vi "Disabled.vi"(7 "Robot Mode":T2, 10 "Match Info":T1={"Autonomous Elapsed Seconds"=0.0, "TeleOp Elapsed Seconds"=0.0, "Disabled Elapsed Seconds"=0.0, "Visited Autonomous"=FALSE, "Visited TeleOp"=FALSE, "Visited Disabled"=FALSE, "Autonomous Settings"={"Autonomous Style"=enum."Independent", "VI Refnum"=refnum}}, 11 "Call Context":T3) -> ()   [LabVIEW 2014]
doc: "This VI is called each time a disabled packet is received from the DS. It is often used to prepare for the next robot mode, to calibrate sensors, etc."
uses:
  <vilib>/Rock Robotics/WPI/DriverStation/WPI_DriverStationDerivedRobotMode.ctl
  <vilib>/Rock Robotics/WPI/DriverStation/WPI_DriverStationRobotMode2.ctl
  <vilib>/Rock Robotics/WPI/DriverStation/WPI_DriverStationMatch Info.ctl
  Elevator System/Elevator System.lvlib
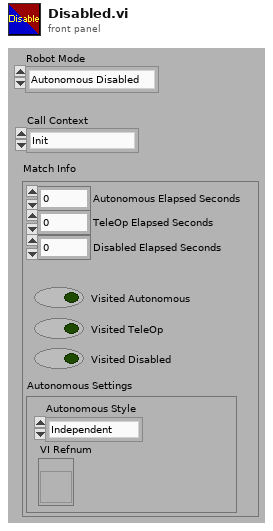
[diagram p1: front panel]
types:
  T1 = typedef "WPI_DriverStationMatch Info.ctl" = cluster{"Autonomous Elapsed Seconds":dbl, "TeleOp Elapsed Seconds":dbl, "Disabled Elapsed Seconds":dbl, "Visited Autonomous":bool, "Visited TeleOp":bool, "Visited Disabled":bool, "Autonomous Settings":cluster{"Autonomous Style":enum16{"Iterative", "Independent"}, "VI Refnum":refnum<vi>}}
  T2 = typedef "WPI_DriverStationRobotMode2.ctl" = enum16{"Autonomous Disabled", "Autonomous Enabled", "Teleop Disabled", "Teleop Enabled", "Disconnected", "Finish", "Test Disabled", "Test Enabled", "Emergency Stopped"}
  T3 = typedef "WPI_DriverStationDerivedRobotMode.ctl" = enum16{"Init", "Execute", "Stop"}
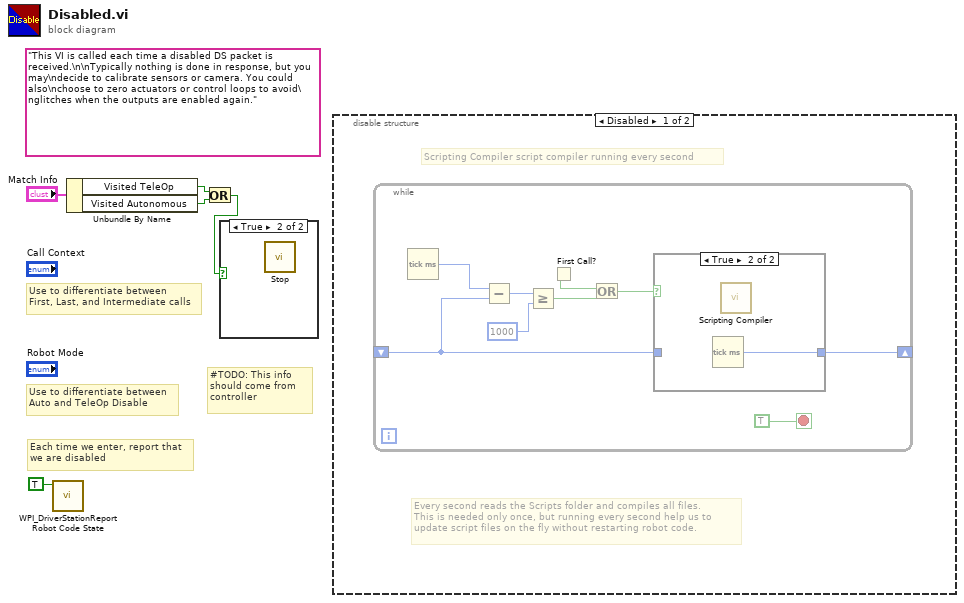
[diagram p0: block diagram]
diagram:
  (unwired) "This VI is called each time a disabled DS packet is received.\n\nTypically nothing is done in response, but you may\ndecide to calibrate sensors or camera. You could also\nchoose to zero actuators or control loops to avoid\nglitches when the outputs are enabled again."
  # "#TODO: This info\nshould come from \ncontroller"
  # "Each time we enter, report that\nwe are disabled"
  # "Use to differentiate between\nFirst, Last, and Intermediate calls"
  # "Use to differentiate between\nAuto and TeleOp Disable"
  n1 = call <vilib>:"WPI_DriverStationReport Robot Code State.vi"("Disabled"=TRUE ("Autonomous")) -> ()  [unwired: 10 in, 1 out]
  n2 = Unbundle By Name("Match Info") -> ("Visited TeleOp"=w3:bool, "Visited Autonomous"=w2:bool)
  n3 = Or(x=w3, y=w2) -> (x .or. y?=w1:bool)
  n4 = case shown="True" w1 {
    frame False {
    }
    frame True {
      n5 = call "Stop.vi"() -> ()  [unwired: 12 in]
    }
  }
  n6 = disable-structure shown="Disabled" {
    frame Disabled {
      # "Every second reads the Scripts folder and compiles all files.\nThis is needed only once, but running every second help us to\nupdate script files on the fly without restarting robot code."
      # "Scripting Compiler script compiler running every second"
      n7 = while {
        shift-right: [w10] -> _
        shift-left: _ -> [w9]
        stop <- TRUE stop-if-true
        n8 = Tick Count (ms)() -> (millisecond timer value=w11:u32)
        n9 = Subtract(x=w11, y=w9) -> (x-y=w13:u32)
        n10 = Greater Or Equal?(x=w13, y=u32 1000) -> (x >= y?=w7:bool)
        n11 = First Call?() -> (First Call?: T/F=w6:bool)
        n12 = Or(x=w6, y=w7) -> (x .or. y?=w8:bool)
        n13 = case shown="True" w8 {
          tunnel: [w15 w16] -> w10
          tunnel: w9 -> [w15 _]
          frame False {
          }
          frame True {
            n14 = Tick Count (ms)() -> (millisecond timer value=w16:u32)
            n15 = call "Scripting Compiler.vi"() -> ()  [unwired: 12 in]
          }
        }
      }
    }
    frame Enabled {
    }
  }
